vi "Untitled 1.vi"() -> ()   [LabVIEW 2018]
uses:
  <vilib>/Utility/file.llb/Read Delimited Spreadsheet (string).vi
panel:
  out "Status":bool[](array[boolean])
  out "Item Names":string[][](array[string])
  out "Numeric 2":i32
  out "Numeric":i32
  out "ItemNames":string[](array[string])
  in  "Device List":i32(listbox)
  in  "Stop":bool
  in  "Config":bool
  in  "EditList":bool
  in  "Tab Control":enum32{"Temp", "RH"}(tab)
  out "TempArray":cluster{"Temp":dbl[][]}[](array[cluster]) caption="ESP32 DEV"
  out "RHArray":cluster{"RH":dbl[][]}[](array[cluster]) caption="ESP32 DEV"
  in  "Liste":path
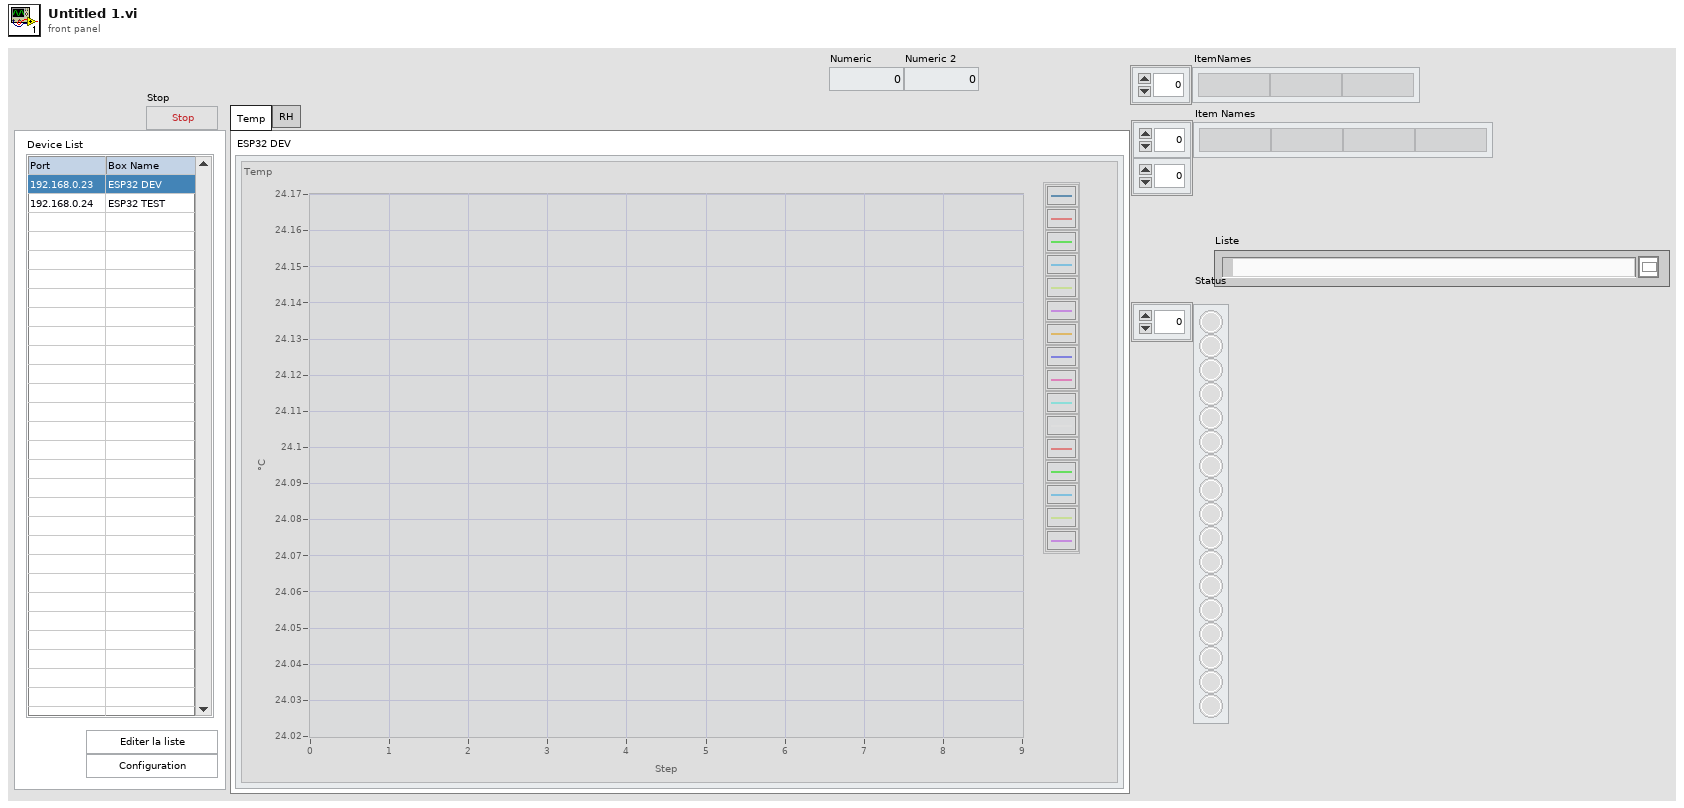
[diagram p1: front panel]
types:
  T1 = cluster{"boxName":string, "SHT-Type":string, "nbSHT":dbl, "version":string}
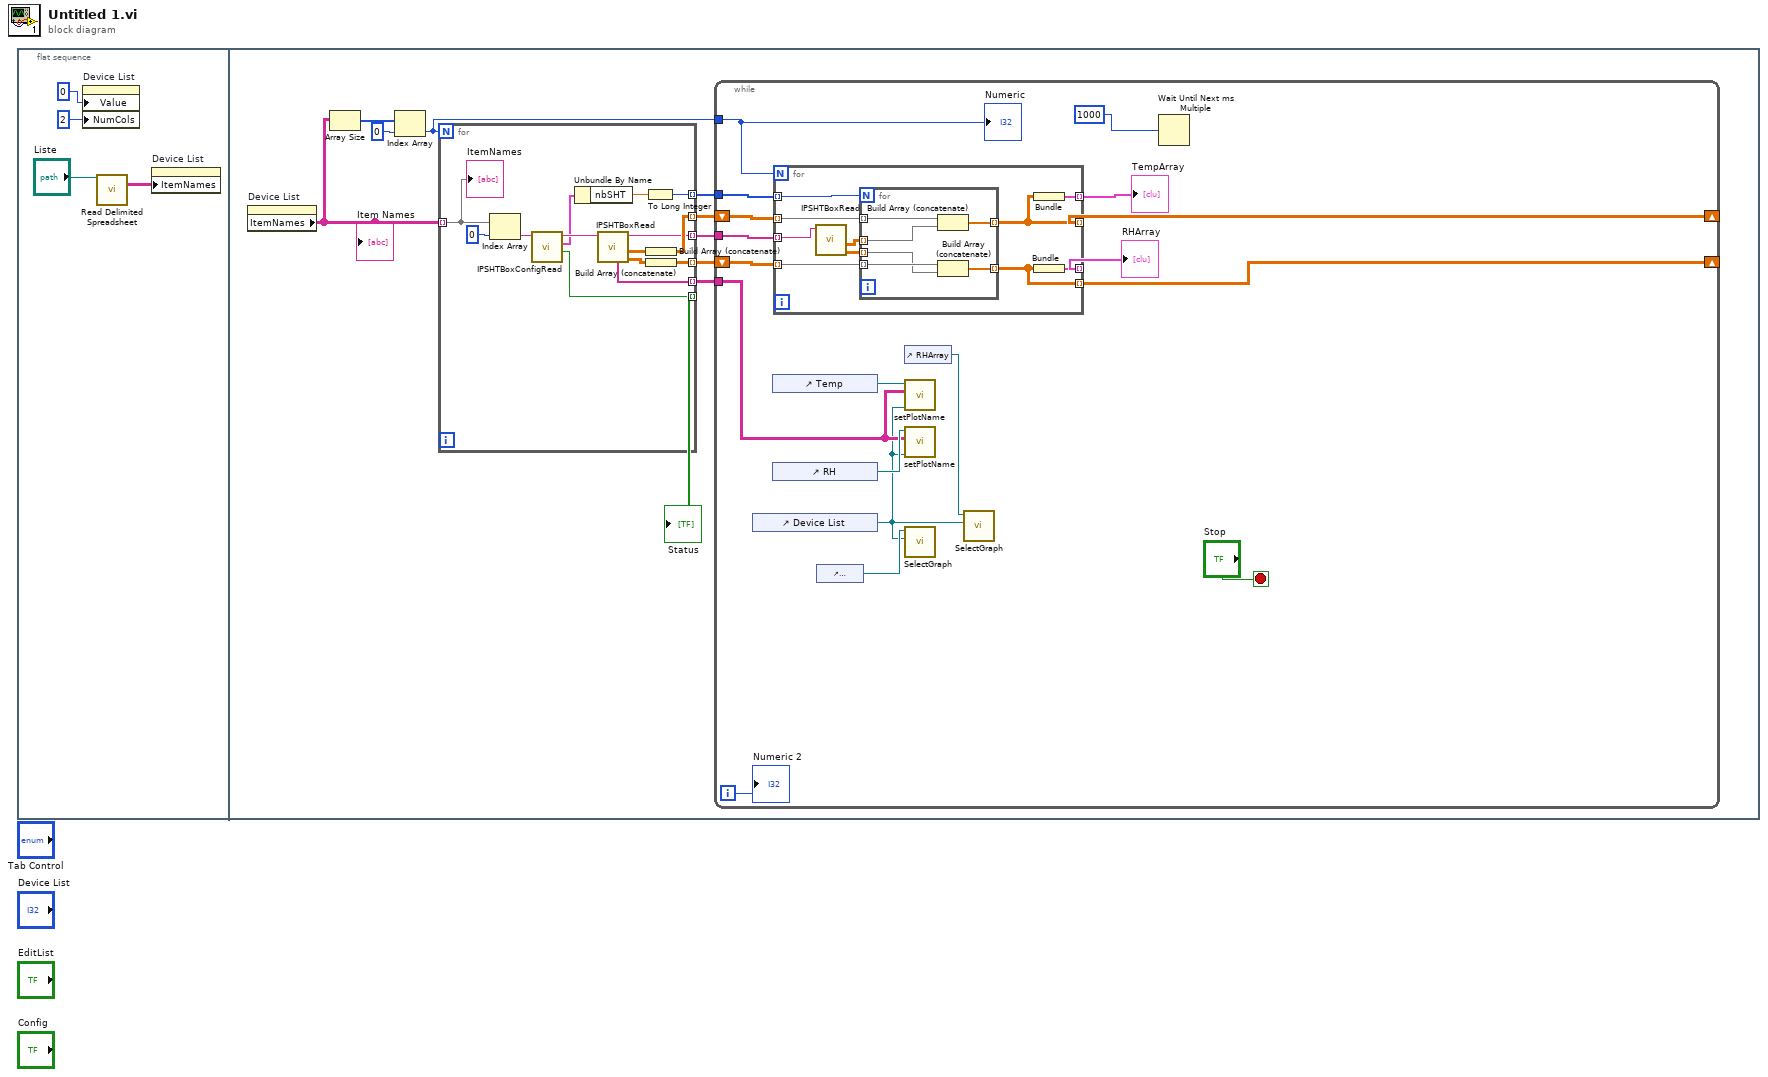
[diagram p0: block diagram]
diagram:
  n1 = flat-sequence {
    frame #0 {
      n2 = property on="Device List" class="MCListbox (strict)"("Value"=0 ("Active Row:Active Row Number"), "NumCols"=u32 2 ("Number of Columns")) -> ()  [unwired: 2 in, 2 out]
      n3 = call-poly <vilib>:"Read Delimited Spreadsheet.vi"("file path (dialog if empty)"="Liste") -> ("all rows"=w4:string[][])  [unwired: 9 in, 5 out]
      n4 = property on="Device List" class="MCListbox (strict)"("ItemNames"=w4) -> ()  [unwired: 2 in, 2 out]
    }
    frame #1 {
      n5 = property on="Device List" class="MCListbox (strict)"() -> ("ItemNames"=w6:string[][])  [unwired: 2 in, 2 out]
      "Item Names" <- w6
      n6 = Array Size(array=w6) -> (size(s)=w9:i32[])
      n7 = Index Array(array=w9, index=0) -> (element=w7:i32)
      n8 = for {
        N: w7 -> [_]
        tunnel: [w28] -> w14 mode=indexing
        tunnel: [w27] -> w13 mode=indexing
        tunnel: [w26] -> w12 mode=indexing
        tunnel: [w25] -> w11 mode=indexing
        tunnel: w6 -> [w24] mode=indexing
        tunnel: [w21] -> w10 mode=indexing
        tunnel: [w15] -> w5 mode=indexing
        n9 = Index Array(array=w24, index=0) -> (element=w22:string)
        n10 = call "IPSHTBoxConfigRead.vi"("IP in"=w22) -> ("status"=w15:bool, "config 2"=w16:T1, "IP out"=w17:string)  [unwired: 7 in, 1 out]
        n11 = Unbundle By Name(w16) -> ("nbSHT"=w19:dbl)
        n12 = call "IPSHTBoxRead.vi"("IP in"=w17) -> ("RH2D"=w18:dbl[][], "Temp2D"=w20:dbl[][], "IP out"=w21:string, "SHTListName"=w27:string[])  [unwired: 5 in, 2 out]
        n13 = To Long Integer(number=w19) -> (32bit integer=w26:i32)
        n14 = Build Array (concatenate)(w20) -> (w28:dbl[][])
        n15 = Build Array (concatenate)(w18) -> (w25:dbl[][])
        "ItemNames" <- w24
      }
      "Status" <- w5
      n16 = while {
        tunnel: w12 -> [w46]
        shift-right: [w44] -> _
        shift-left: w14 -> [w45]
        tunnel: w13 -> [w36]
        shift-right: [w33] -> _
        shift-left: w11 -> [w34]
        tunnel: w10 -> [w31]
        tunnel: w7 -> [w30]
        i -> [w29]
        stop <- "Stop" stop-if-true
        n17 = control-ref of="Device List"() -> (w35:refnum<vi>)
        n18 = control-ref of="Temp"() -> (w39:refnum<vi>)
        n19 = control-ref of="RH"() -> (w38:refnum<vi>)
        n20 = for {
          N: w30 -> [_]
          tunnel: w45 -> [w54] mode=indexing
          tunnel: [w56] -> w43 mode=indexing
          tunnel: w46 -> [w55] mode=indexing
          tunnel: [w53] -> w44 mode=indexing
          tunnel: w34 -> [w51] mode=indexing
          tunnel: [w49] -> w33 mode=indexing
          tunnel: [w48] -> w32 mode=indexing
          tunnel: w31 -> [w47] mode=indexing
          n21 = call "IPSHTBoxRead.vi"("IP in"=w47) -> ("RH2D"=w50:dbl[][], "Temp2D"=w52:dbl[][])  [unwired: 5 in, 4 out]
          n22 = for {
            N: w55 -> [_]
            tunnel: w54 -> [w62] mode=indexing
            tunnel: [w61] -> w53 mode=indexing
            tunnel: w52 -> [w60] mode=indexing
            tunnel: w51 -> [w59] mode=indexing
            tunnel: w50 -> [w58] mode=indexing
            tunnel: [w57] -> w49 mode=indexing
            n23 = Build Array (concatenate)(w62, w60) -> (w61:dbl[])
            n24 = Build Array (concatenate)(w59, w58) -> (w57:dbl[])
          }
          n25 = Bundle(w53) -> (w56:cluster{dbl[][]})  [unwired: 1 in]
          n26 = Bundle(w49) -> (w48:cluster{dbl[][]})  [unwired: 1 in]
        }
        "TempArray" <- w43
        "RHArray" <- w32
        n27 = control-ref of="TempArray"() -> (w41:refnum<vi>)
        n28 = control-ref of="RHArray"() -> (w40:refnum<vi>)
        n29 = call "setPlotName.vi"("reference"=w35, "Array"=w36, "WaveformGraph in"=w39) -> ()  [unwired: 9 in]
        n30 = call "setPlotName.vi"("reference"=w35, "Array"=w36, "WaveformGraph in"=w38) -> ()  [unwired: 9 in]
        n31 = call "SelectGraph.vi"("reference"=w35, "Array in"=w41) -> ()  [unwired: 10 in]
        n32 = call "SelectGraph.vi"("reference"=w35, "Array in"=w40) -> ()  [unwired: 10 in]
        n33 = Wait Until Next ms Multiple(millisecond multiple=u32 1000) -> ()  [unwired: 1 out]
        "Numeric" <- w30
        "Numeric 2" <- w29
      }
    }
  }
